vi "Data Cluster Plotter.vi"() -> (0 "output cluster":T2)   [LabVIEW 2013]
uses:
  plotter setup cluster.ctl
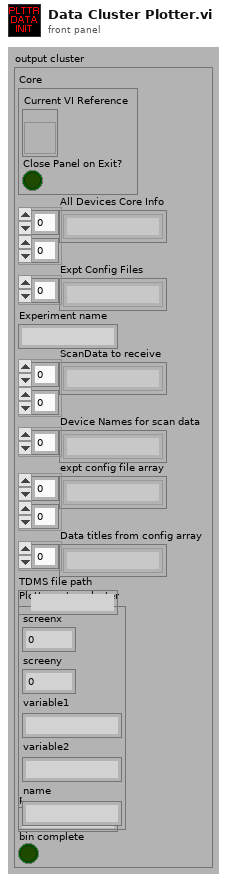
[diagram p1: front panel]
types:
  T1 = typedef "plotter setup cluster.ctl" = cluster{"screenx":i16, "screeny":i16, "variable1":string, "variable2":string, "name":string}
  T2 = cluster{"Core":cluster{"Current VI Reference":refnum<vi>, "Close Panel on Exit?":bool}, "All Devices Core Info":string[][], "Expt Config Files":string[], "Experiment name":string, "ScanData to receive":string[][], "Device Names for scan data":string[], "expt config file array":string[][], "Data titles from config array":string[], "TDMS file path":path, "Plotter setup cluster":T1, "plotter#":string, "bin complete":bool}
  T3 = cluster{"Current VI Reference":refnum<vi>, "Close Panel on Exit?":bool}
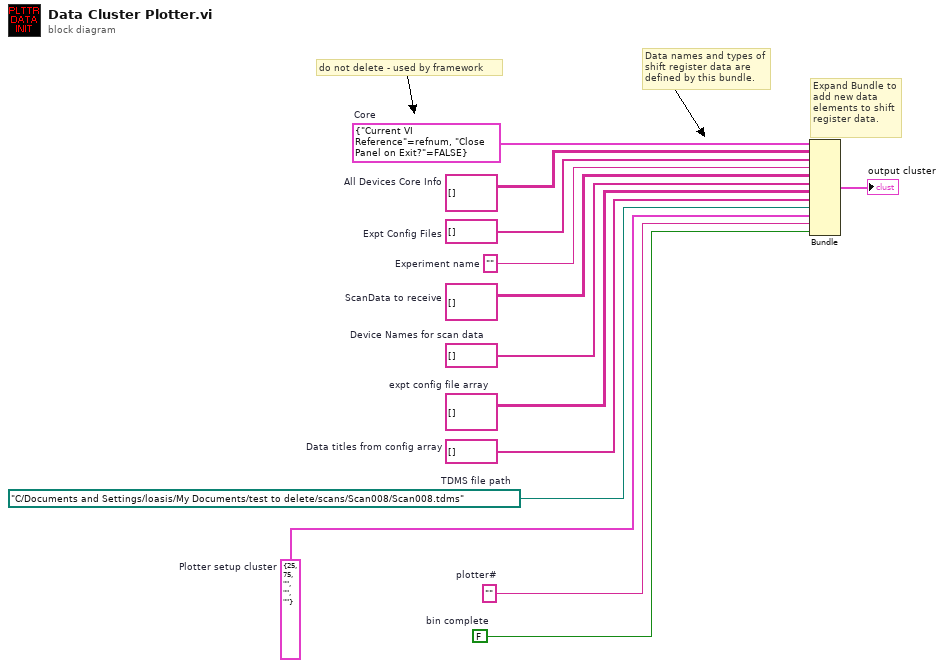
[diagram p0: block diagram]
diagram:
  w2 = FALSE  # bin complete
  w3 = ""  # plotter#
  w4 = T1 {"screenx"=25, "screeny"=75, "variable1"="", "variable2"="", "name"=""}  # Plotter setup cluster
  w5 = path "C:/Documents and Settings/loasis/My Documents/test to delete/scans/Scan008/Scan008.tdms"  # TDMS file path
  w6 = string[] []  # Data titles from config array
  w7 = string[][] []  # expt config file array
  w8 = string[] []  # Device Names for scan data
  w9 = string[][] []  # ScanData to receive
  w10 = ""  # Experiment name
  w11 = string[] []  # Expt Config Files
  w13 = string[][] []  # All Devices Core Info
  w12 = T3 {"Current VI Reference"=refnum, "Close Panel on Exit?"=FALSE}  # Core
  # "do not delete - used by framework"
  # "Expand Bundle to add new data elements to shift register data."
  # "Data names and types of shift register data are defined by this bundle."
  n1 = Bundle("Core"=w12, "All Devices Core Info"=w13, "Expt Config Files"=w11, "Experiment name"=w10, "ScanData to receive"=w9, "Device Names for scan data"=w8, "expt config file array"=w7, "Data titles from config array"=w6, "TDMS file path"=w5, "Plotter setup cluster"=w4, "plotter#"=w3, "bin complete"=w2) -> (→"output cluster":T2)  [unwired: 1 in]
